vi "Read HIL Data and Write to Shared Variable.vi"(8 "error in":errorcluster) -> (0 "error out":errorcluster)   [LabVIEW 2017, in "DTACQ - Network Enabled Device Driver.lvlib"]
uses:
  DTACQ - Network Enabled Device Driver.lvlib
  Communications/Typedefs/Functional Global Variable Action--Enum.ctl
  FGV Operaions--Enum.ctl
  Network Shared Variables/Typedefs/X and Y Variant Arrays--Cluster.ctl
  Communications/Communications Library.lvlib
  Network Shared Variables/Shared Variables Library.lvlib
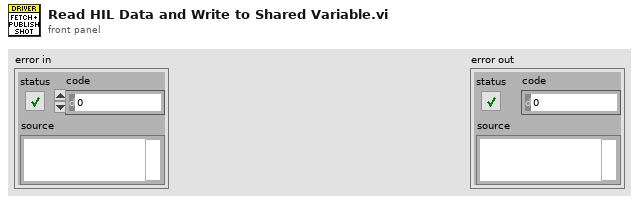
[diagram p1: front panel]
types:
  T1 = typedef "DTACQ - Network Enabled Device Driver.lvlib/FGV Operaions--Enum.ctl" = enum16{"Get Driver Settings", "Set Driver Settings", "Search Variable Names", "Close Connections", "Open Connections", "Get Variable References", "Set Variable References", "Clear"}
  T2 = typedef "Communications Library.lvlib/Functional Global Variable Action--Enum.ctl" = enum16{"Initialise", "Write Module Config", "Write Carrier Config", "Read"}
  T3 = typedef "Communications Library.lvlib/DTACQ Module Carrier Configuration--Cluster.ctl" = cluster{"Name":string, "IP":string, "Control Port":i32, "Timeout (ms)":i32, "Continuous Capture Port (Multiplexed)":i32, "Start HIL Shot Port":i32, "AWG Upload Port (Multiplexed)":i32, "Download Captured Data Port (Multiplexed)":i32, "Module Slots":i32, "Module Configurations":T4[]}
  T4 = typedef "Communications Library.lvlib/DTACQ Module Configuration--Cluster.ctl" = cluster{"Name":string, "Position":string, "Module Type":T5, "Control Port":i32, "Timeout (ms)":i32, "Channels":i32}
  T5 = typedef "Communications Library.lvlib/DTACQ Device Type--Enum.ctl" = enum16{"Carrier", "Analog In Module", "Analog Out Module", "Generic Module"}
  T6 = typedef "DTACQ - Network Enabled Device Driver.lvlib/Driver Global Settings--Typedef.ctl" = cluster{"Waveform Length":i32, "Data Size":T7, "DTACQ Connection Data":T8}
  T7 = typedef "Communications Library.lvlib/Data Size--Enum.ctl" = enum16{"16 Bit (Signed Short)", "32 Bit (Signed Long)"}
  T8 = typedef "Communications Library.lvlib/DTACQ Connection Data--Cluster.ctl" = cluster{"Description":string, "Address":string, "Port":u16, "timeout (ms)":i32, "Termination Character":string, "TCP Connection Reference":refnum<k5>, "Open Connection":bool}
  T9 = typedef "Shared Variables Library.lvlib/X and Y Variant Arrays--Cluster.ctl" = cluster{"X-Data":variant[], "Y-Data":variant[]}
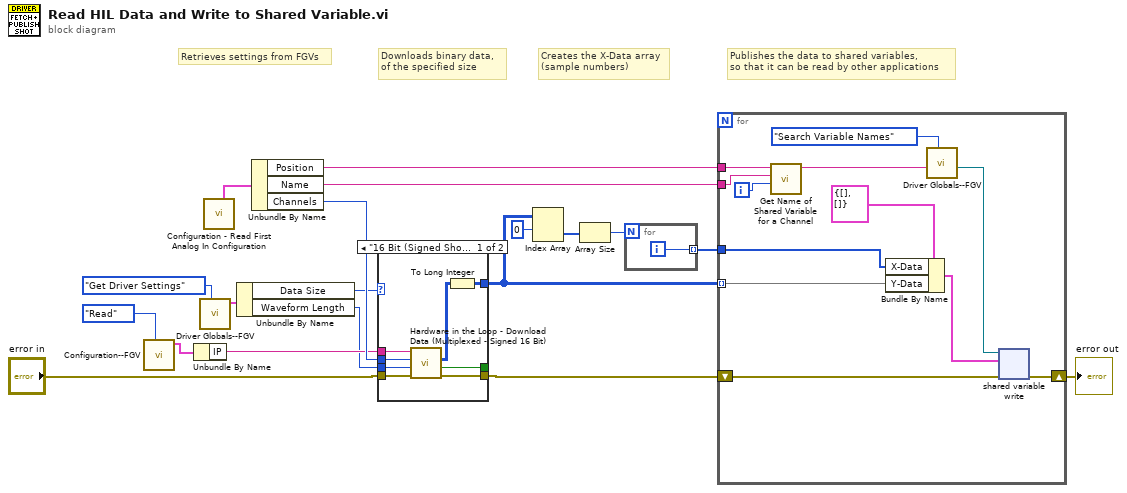
[diagram p0: block diagram]
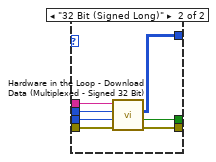
[diagram p2: hidden frame]
diagram:
  # "Publishes the data to shared variables,\nso that it can be read by other applications"
  # "Creates the X-Data array\n(sample numbers)"
  # "Downloads binary data,\nof the specified size"
  # "Retrieves settings from FGVs"
  n1 = call "Configuration--FGV.vi"("Functional Global Action"=Functional_Global_Variable_Action--Enum."Read") -> ("Carrier Configuration Out"=w18:T3)  [unwired: 9 in, 1 out]
  n2 = Unbundle By Name(w18) -> ("IP"=w14:string)
  n3 = call "Driver Globals--FGV.vi"(7:FGV_Operaions--Enum."Get Driver Settings") -> ("Driver Settings Out"=w6:T6)  [unwired: 7 in, 3 out]
  n4 = call "Configuration - Read First Analog In Configuration.vi"() -> ("AI - Module Configuration"=w16:T4)  [unwired: 7 in, 4 out]
  n5 = Unbundle By Name(w6) -> ("Data Size"=w1:T7, "Waveform Length"=w5:i32)
  n6 = Unbundle By Name(w16) -> ("Position"=w8:string, "Name"=w7:string, "Channels"=w15:i32)
  n7 = case shown="\"16 Bit (Signed Short)\", Default" w1 {
    tunnel: w15 -> [w27 w29]
    tunnel: w5 -> [w26 w28]
    tunnel: [w25 w33] -> w3
    tunnel: w14 -> [w24 w30]
    tunnel: "error in" -> [w23 w34]
    tunnel: [w22 w32] -> _
    tunnel: [w20 w31] -> w12
    frame "16 Bit (Signed Short)", Default {
      n8 = call "Hardware in the Loop - Download Data (Multiplexed - Signed 16 Bit).vi"("error in"=w23, "Number of Samples"=w26, "Number of Channels"=w27, "Address"=w24) -> ("error out"=w25:errorcluster, "Data Received"=w22:bool, "Data"=w21:i16[][])  [unwired: 5 in]
      n9 = To Long Integer(number=w21) -> (32bit integer=w20:i32[][])
    }
    frame "32 Bit (Signed Long)" {
      n10 = call "Hardware in the Loop - Download Data (Multiplexed - Signed 32 Bit).vi"("error in"=w34, "Number of Samples"=w28, "Number of Channels"=w29, "Address"=w30) -> ("error out"=w33:errorcluster, "Data Received"=w32:bool, "Data"=w31:i32[][])  [unwired: 5 in]
    }
  }
  n11 = Index Array(array=w12, index (row)=0) -> (element=w10:i32[])  [unwired: 1 in]
  n12 = Array Size(array=w10) -> (size(s)=w13:i32)
  n13 = for {
    N: w13 -> [_]
    tunnel: [w35] -> w9 mode=indexing
    i -> [w35]
  }
  n14 = for {
    tunnel: w12 -> [w46] mode=indexing
    tunnel: w9 -> [w45]
    tunnel: w8 -> [w44]
    tunnel: w7 -> [w43]
    shift-right: [w36] -> w2
    shift-left: w3 -> [w37]
    i -> [w47]
    n15 = call "Get Name of Shared Variable for a Channel.vi"("Channel Number"=w47, "Module Name"=w43, "Module Position"=w44) -> ("Shared Variable Name"=w40:string)  [unwired: 8 in]
    n16 = Bundle By Name(cluster=T9 {"X-Data"=[], "Y-Data"=[]} ("Data Cluster"), "X-Data"=w45, "Y-Data"=w46) -> (w38:T9)
    n17 = call "Driver Globals--FGV.vi"(7:FGV_Operaions--Enum."Search Variable Names", "Name"=w40) -> ("Searched Reference"=w39:refnum<k21>)  [unwired: 6 in, 3 out]
    n18 = shared-variable-write(w39, w37, w38) -> (w36:errorcluster)  [unwired: 1 out]
  }
  "error out" <- w2
